vi "WAA.vi"(0 "System no.":i32=1 min=1 max=4 step=1, 3 "Timeout, ms":i32=500 min=1 max=4 step=1, 5 "error in":errorcluster, 12 "Stop refnum":refnum<vi>) -> (14 "Ready?":bool, 19 "error out":errorcluster)   [LabVIEW 2020]
doc: "Wait for all axes with timeout. This VI returns as soon as the movement of all connected axes has finished, Local stop or Stop refnum is TRUE or after the specified timeout has elapsed. It returns Ready? = TRUE if motion was completed, Ready? = FALSE if timeout elapsed or VI was stopped. When using as a sub-VI, use Stop refnum to stop VI from caller."
panel:
  in  "Local stop":bool
  # "Wait for all axes with timeout."
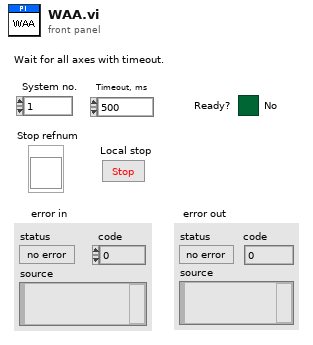
[diagram p1: front panel]
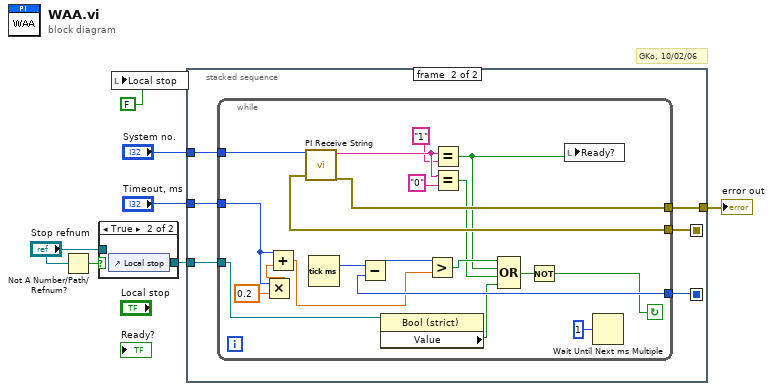
[diagram p0: block diagram]
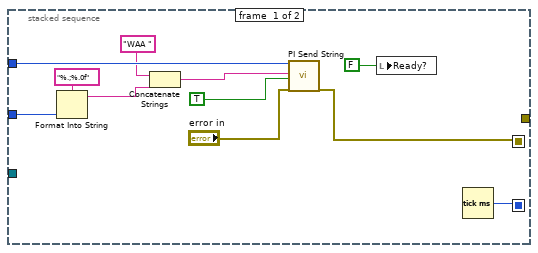
[diagram p3: hidden frame]
diagram:
  # "GKo, 10/02/06"
  n1 = Not A Number/Path/Refnum?(number/path/refnum="Stop refnum") -> (NaN/Path/Refnum?=w2:bool)
  n2 = case shown="True" w2 {
    tunnel: [w8 w9] -> w1
    tunnel: "Stop refnum" -> [w8 _]
    frame False {
    }
    frame True {
      n3 = control-ref of="Local stop"() -> (w9:refnum<vi>)
    }
  }
  n4 = local write "Local stop"(FALSE ("Local stop")) -> ()
  n5 = stacked-sequence {
    seq-local: [w19 _] -> [_ w26]
    seq-local: [w15 _] -> [_ w24]
    tunnel: "System no." -> [w16 w25]
    tunnel: [_ w23] -> w6
    tunnel: "Timeout, ms" -> [w14 w22]
    tunnel: w1 -> [_ w21]
    frame #0 {
      n6 = Format Into String(format string="%.;%.0f" ("Format String"), w14) -> (resulting string=w13:string)  [unwired: 2 in, 1 out]
      n7 = Concatenate Strings("WAA ", w13) -> (w11:string)
      n8 = call "PI Send String.vi"("System no."=w16, "String to send"=w11, "Attach termination char.?"=TRUE ("Attach Linefeed?"), "error in"="error in") -> ("error out"=w19:errorcluster)  [unwired: 15 out]
      n9 = local write "Ready?"(FALSE ("Moving?")) -> ()
      n10 = Tick Count (ms)() -> (millisecond timer value=w15:u32)
    }
    frame #1 {
      n11 = while {
        tunnel: w21 -> [w30]
        tunnel: w22 -> [w33]
        tunnel: [w38] -> w23
        tunnel: w24 -> [w44]
        tunnel: w25 -> [w46]
        tunnel: w26 -> [w47]
        stop <- w40 continue-if-true
        n12 = Multiply(x=w33, y=0.2) -> (x*y=w31:dbl)
        n13 = Add(x=w33, y=w31) -> (x+y=w36:dbl)
        n14 = call "PI Receive String.vi"("System no."=w46, "error in"=w47) -> ("String read"=w35:string, "error out"=w38:errorcluster)  [unwired: 1 in, 15 out]
        n15 = Tick Count (ms)() -> (millisecond timer value=w45:u32)
        n16 = Subtract(x=w45, y=w44) -> (x-y=w43:u32)
        n17 = property class="Bool (strict)"(reference=w30) -> ("Value"=w29:bool)  [unwired: 1 in, 2 out]
        n18 = Greater?(x=w43, y=w36) -> (0:w42:bool)
        n19 = Equal?(x=w35, y="1") -> (x = y?=w37:bool)
        n20 = Equal?(x=w35, y="0") -> (x = y?=w34:bool)
        n21 = Compound Arithmetic op=OR(w42, w37, w34, w29) -> (w41:bool)
        n22 = Not(x=w41) -> (.not. x?=w40:bool)
        n23 = local write "Ready?"(w37) -> ()
        n24 = Wait Until Next ms Multiple(millisecond multiple=u32 1) -> ()  [unwired: 1 out]
      }
    }
  }
  "error out" <- w6
